vi "call restart.vi"(8 "error in (no error)":errorcluster) -> (0 "error out":errorcluster)   [LabVIEW 2015]
uses:
  <vilib>/Utility/config.llb/Write Key (String).vi
  <vilib>/Utility/config.llb/NI_LVConfig.lvlib
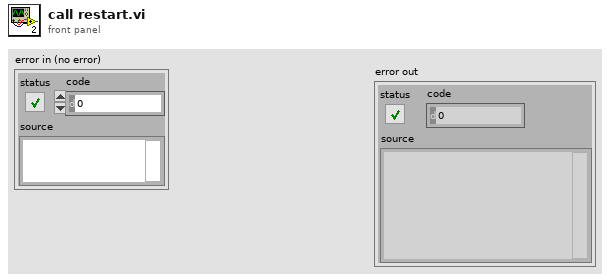
[diagram p1: front panel]
types:
  T1 = typedef "NI_LVConfig.lvlib/Config Data RefNum.ctl" = refnum<k1>
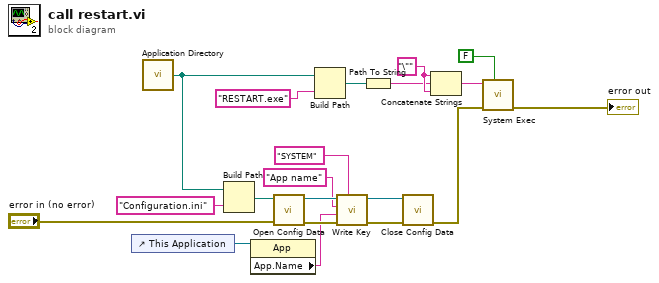
[diagram p0: block diagram]
diagram:
  w16 = "\""
  n1 = control-ref of="This Application"() -> (w4:refnum<vi>)
  n2 = call <vilib>:"Application Directory.vi"() -> ("Application Directory"=w10:path)
  n3 = Build Path(base path=w10, name or relative path="Configuration.ini") -> (appended path=w11:path)
  n4 = property class="App"(reference=w4) -> ("App.Name"=w1:string)  [unwired: 1 in, 2 out]
  n5 = call <vilib>:"Open Config Data.vi"("error in (no error)"="error in (no error)", "configuration file path"=w11) -> ("error out"=w8:errorcluster, "refnum"=w12:T1)  [unwired: 7 in, 1 out]
  n6 = Build Path(base path=w10, name or relative path="RESTART.exe") -> (appended path=w17:path)
  n7 = call-poly <vilib>:"Write Key.vi"("section"="SYSTEM", "error in (no error)"=w8, "value"=w1, "key"="App name", "refnum"=w12) -> ("error out"=w7:errorcluster, "refnum out"=w13:T1)  [unwired: 4 in, 1 out]
  n8 = Path To String(path=w17) -> (string=w15:string)
  n9 = call <vilib>:"Close Config Data.vi"("error in (no error)"=w7, "refnum"=w13) -> ("error out"=w3:errorcluster)  [unwired: 8 in, 1 out]
  n10 = Concatenate Strings(w16, w15, w16) -> (w20:string)
  n11 = call <vilib>:"System Exec.vi"("wait until completion? (T)"=FALSE, "error in (no error)"=w3, "command line"=w20) -> ("error out"=→"error out":errorcluster)  [unwired: 5 in, 3 out]
